vi "N6(problem).vi"() -> ()   [LabVIEW 2020]
uses:
  7f9115e3-b111-487f-af19-15bf33eaf760.vi
  <vilib>/Comparison/Less/Less Functor/Less Functor.lvclass
panel:
  out "array":dbl[](array[numeric])
  out "Sort":string
  out "error out":errorcluster
  in  "file path (use dialog)":path
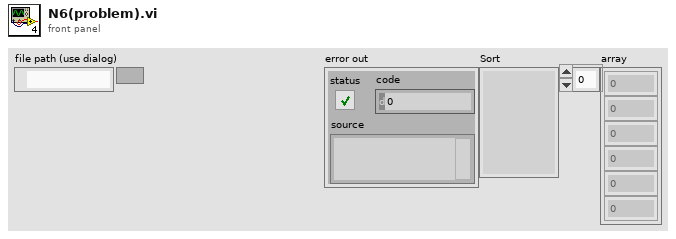
[diagram p1: front panel]
types:
  T1 = enum16{"open", "replace", "create", "open or create", "replace or create", "replace or create with confirmation"}
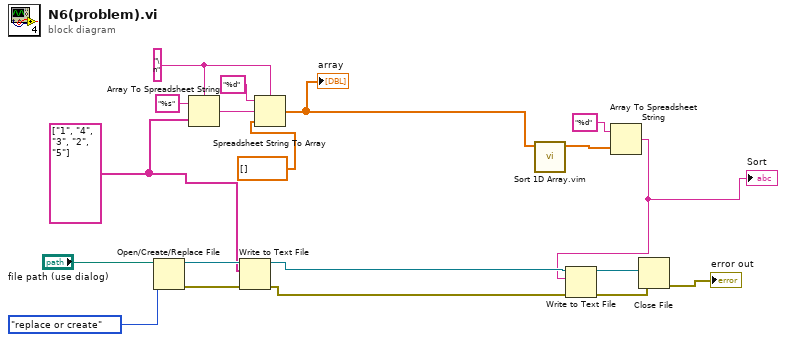
[diagram p0: block diagram]
diagram:
  w4 = "\n" ("delimiter (Tab)")
  w7 = string[] ["1", "4", "3", "2", "5"]
  n1 = Open/Create/Replace File(file path (use dialog)="file path (use dialog)", operation (0:open)=T1."replace or create") -> (refnum out=w18:refnum<file>, error out=w17:errorcluster)  [unwired: 4 in, 1 out]
  n2 = Array To Spreadsheet String(delimiter (Tab)=w4, array=w7, 3:"%s" ("format string")) -> (spreadsheet string=w5:string)
  n3 = Write to Text File(file (use dialog)=w18, text=w7, error in=w17) -> (refnum out=w12:refnum<file>, error out=w11:errorcluster)  [unwired: 1 in, 1 out]
  n4 = Spreadsheet String To Array(delimiter (Tab)=w4, format string="%d", spreadsheet string=w5, array type (2D Dbl)=dbl[] []) -> (array=w1:dbl[])
  "array" <- w1
  n5 = call "Sort 1D Array.vim"("unsorted array"=w1) -> ("sorted array"=w9:dbl[])  [unwired: 10 in]
  n6 = Array To Spreadsheet String(array=w9, 3:"%d" ("format string")) -> (spreadsheet string=w8:string)  [unwired: 1 in]
  "Sort" <- w8
  n7 = Write to Text File(file (use dialog)=w12, text=w8, error in=w11) -> (refnum out=w15:refnum<file>, error out=w14:errorcluster)  [unwired: 1 in, 1 out]
  n8 = Close File(refnum=w15, error in=w14) -> (error out=→"error out":errorcluster)  [unwired: 1 out]
